vi "DashboardCloseSafetyPopup.vi"(8 "Dashboard":refnum<k24>, 11 "error in":errorcluster) -> (0 "Response":cluster{"Message":string, "Succeed":bool}, 3 "error out":errorcluster)   [LabVIEW 2016, in "UnderAutomation.UniversalRobots.lvlib"]
uses:
  UnderAutomation.UniversalRobots.lvlib
  C:/Users/fg/Documents/UniversalRobots.vi/LabVIEW_2024/UnderAutomation.UniversalRobots/lib/UnderAutomation.UniversalRobots.dll
  LabVIEW_2024/UnderAutomation.UniversalRobots/lib/UnderAutomation.UniversalRobots.dll
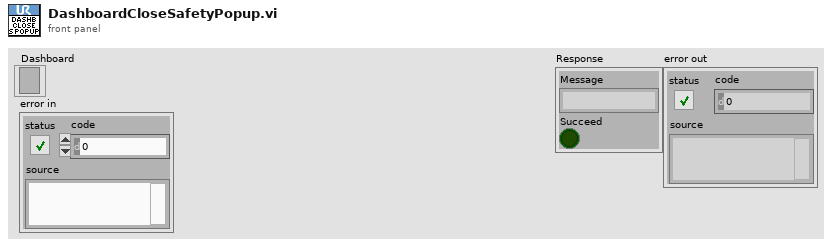
[diagram p1: front panel]
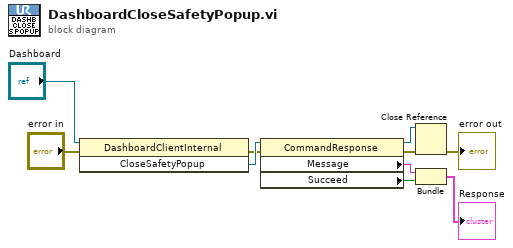
[diagram p0: block diagram]
diagram:
  n1 = invoke class="DashboardClientInternal" method="CloseSafetyPopup"(reference="Dashboard", error in="error in") -> (error out=w4:errorcluster, "CloseSafetyPopup"=w9:refnum<k24>)  [unwired: 1 in, 1 out]
  n2 = property class="CommandResponse"(reference=w9, error in=w4) -> (reference out=w1:refnum<k24>, error out=w3:errorcluster, "Message"=w8:string, "Succeed"=w7:bool)
  n3 = Close Reference(reference=w1, error in (no error)=w3) -> (error out=→"error out":errorcluster)
  n4 = Bundle("Message"=w8, "Succeed"=w7) -> (→"Response":cluster{"Message":string, "Succeed":bool})  [unwired: 1 in]
